vi "THz_TimeDelay.vi"(8 "error in (no error)":errorcluster, 11 "Transport":refnum<class "Transport.lvclass">) -> (0 "error out":errorcluster, 3 "Transport out":refnum<class "Transport.lvclass">)   [LabVIEW 2019, in "Transport.lvclass"]
uses:
  Transport.lvclass
  Transport.lvclass/Transport.ctl
  Control Experiment/Control Experiment.lvclass/Control Experiment.ctl
  <vilib>/PRIrvin/XY Utilities/subVIs/Waveform to XY (single).vi
  <vilib>/PRIrvin/XY Utilities/subVIs/Get X and Y (single).vi
  <userlib>/_MGI/Timing/MGI Wait/MGI Wait (U32).vi
  <vilib>/Waveform/WDTOps.llb/WDT Append Waveforms DBL.vi
  <vilib>/Waveform/WDTOps.llb/Waveform to XY Pairs.vi
  <vilib>/Waveform/WDTOps.llb/WDT Waveform to XY Pairs DBL.vi
  <vilib>/measure/maspectr.llb/FFT Power Spectrum and PSD for 1 Chan.vi
  Control Experiment/Control Experiment.lvclass
  <userlib>/LevyLab/Lockin-Multichannel/Instrument.Lockin/Instrument.Lockin.lvclass
  <userlib>/LevyLab/Instrument Framework/Instrument Types/Delay Line/Instrument.DelayLine.lvclass
  <userlib>/LevyLab/Instrument Framework/Instrument Types/Cryostat/Instrument.Cryostat.lvclass
  <vilib>/measure/NI_MAPro.lvlib
  <vilib>/PRIrvin/XY Utilities/xy_utilities.lvlib
  <userlib>/LevyLab/Instrument Framework/Instrument Types/Lockin/Instrument.LockinAPI.lvclass
  C:/Program Files (x86)/National Instruments/LabVIEW 2019/user.lib/LevyLab/Instrument Framework/Instrument Types/Lockin/Instrument.LockinAPI.lvclass
  C:/Program Files (x86)/National Instruments/LabVIEW 2019/user.lib/LevyLab/Instrument Framework/Instrument/Instrument.lvclass
  C:/Program Files (x86)/National Instruments/LabVIEW 2019/vi.lib/JKI/JKI SMO/SMO/SMO.lvclass
  <vilib>/measure/maresamp.llb/Resample Pair of Arrays (single shot).vi
panel:
  out "Horizontal Progress Bar":dbl(slide)=0.5013000000000001 scale=-0.5..0.5
  out "Signal vs Time":T1(graph)
  out "Delay vs Time":cluster{"Time":dbl[], "Delay":dbl[]}(graph)
  out "Power Spectrum":cluster{"f0":dbl, "df":dbl, "magnitude":dbl[]}[](graph) caption="Power spectrum of time domain signal"
  in  "stop":bool
  in  "Experiment Comments":string="describe only the experiment you're doing right now"
  in  "Experiment Folder":string="05 - folder name"
  out "Delay (ps)":dbl
  out "Elapsed Time (s)":u32
  out "T (mK)":dbl
  out "Refresh Time (ms)":u32
  in  "Sweep Time (s)":dbl=10.0 format="%#_3p"
  in  "Initial Wait (s)":u32=1
  in  "Delay End (ps)":dbl=0.5
  in  "Delay Start (ps)":dbl=-0.5
  in  "Fs (S/s)":dbl=1000.0 min=1000.0 max=204800.0 format="%#_13g"
  in  "Lockin Refresh (s)":dbl=2.0
  in  "Timeout (ms)":i32=1000
  out "Current State":string="Exit"
  # "Start"
  # "End"
  # "*** Folder and comments are only read if this VI is top level. If is is called from Sweep Control then the folder and comments come from Sweep Control.vi ***"
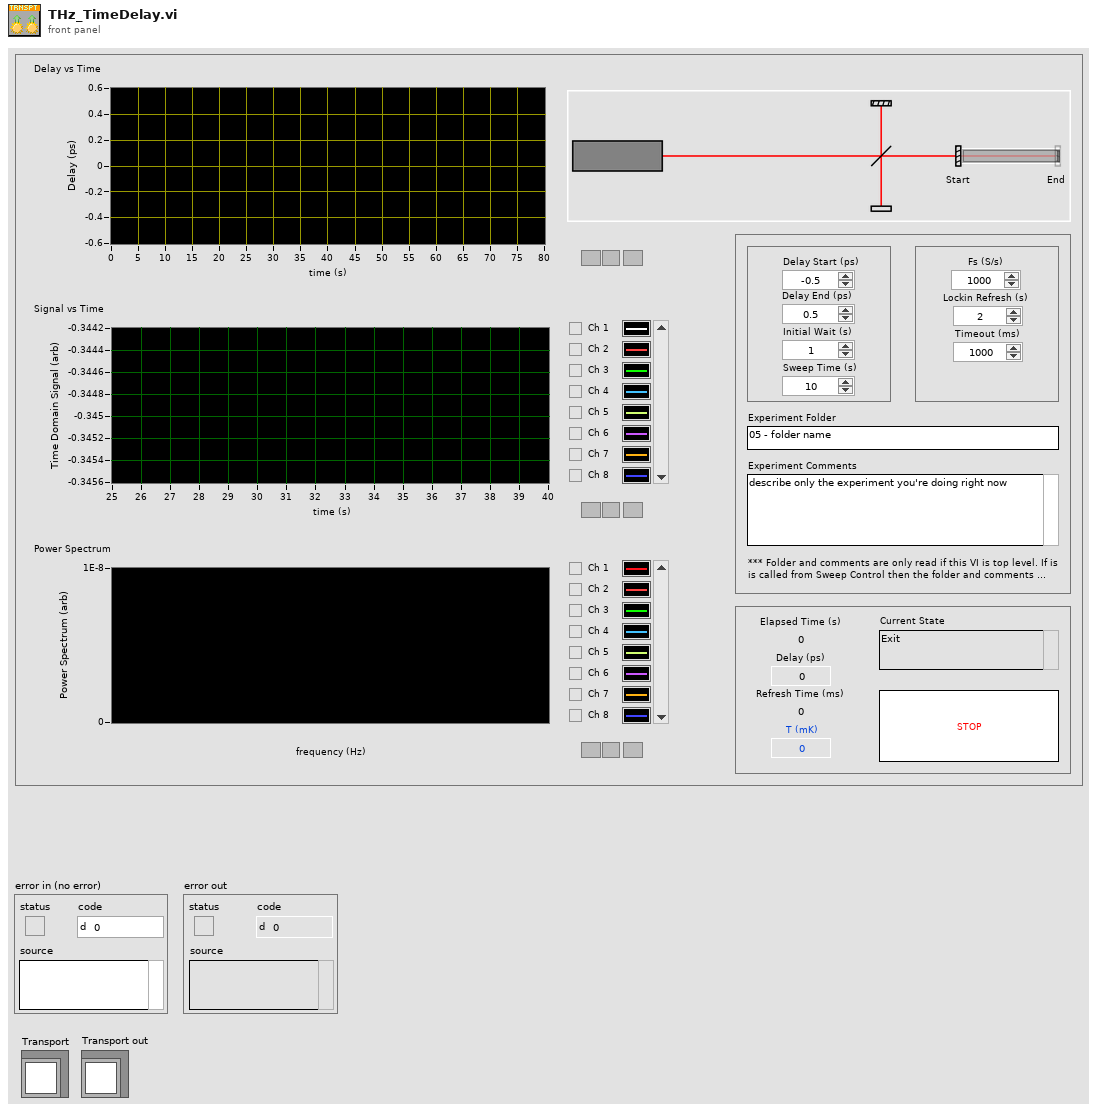
[diagram p1: front panel]
types:
  T1 = cluster{"Delay Start (ps)":dbl, dbl, "Y":dbl[]}[]
  T2 = enum32{"Invalid", "Standard", "Closed", "Hidden", "Minimized", "Maximized"}
  T3 = enum32{"invalid app kind", "Development System", "Run Time System", "Student Edition", "Embedded LabVIEW", "Evaluation", "Custom"}
  T4 = typedef "Control Experiment.lvclass/Instrument Classes--cluster.ctl" = cluster{"DAQ":refnum<class "Instrument.LockinAPI.lvclass">, "Amplifier":refnum<class "Instrument.Amplifier.lvclass">, "Temperature":refnum<class "Instrument.Cryostat.lvclass">, "Magnet":refnum<class "Instrument.Cryostat.lvclass">, "Rotator":refnum<class "Instrument.Cryostat.lvclass">, "Level":refnum<class "Instrument.Cryostat.lvclass">, "Capacitance":refnum<class "Instrument.CBridge.lvclass">, "Delay Line":refnum<class "Instrument.DelayLine.lvclass">, "Strain Cell":refnum<class "Instrument.Strain.lvclass">, "VNA":refnum<class "Instrument.VNA.lvclass">, "Source":refnum<class "Instrument.VSource.lvclass">}
  T5 = cluster{"Core":cluster{"Current VI Reference":refnum<vi>, "Close Panel on Exit?":bool}, "Transport":refnum<class "Transport.lvclass">, "C.E.":refnum<class "Control Experiment.lvclass">, "Instruments":T4, "Elapsed Time":dbl[], "Absolute Time":dbl[], "Temperature":dbl, "Magnet":dbl, "Delay":dbl[], "AI Waveform (s)":waveform(dbl)[], "AI Waveform (ps)":waveform(dbl)[], "t0":timestamp, "Sweep Value":dbl[], "ms [0]":u32, "ms [i]":u32, "Delay Range (ps)":dbl, "Delay Speed (ps/s)":dbl, "reset":bool, "delay line finish?":bool, "Execution:State":enum32{"Bad", "Idle", "Run top level", "Running"}}
  T6 = enum32{"Bad", "Idle", "Run top level", "Running"}
  T7 = cluster{"Current VI Reference":refnum<vi>, "Close Panel on Exit?":bool}
  T8 = typedef "Instrument.LockinAPI.lvclass/LockinAPI.Sampling.Sampling--Cluster.ctl" = cluster{"Fs":dbl, "#s":i32}
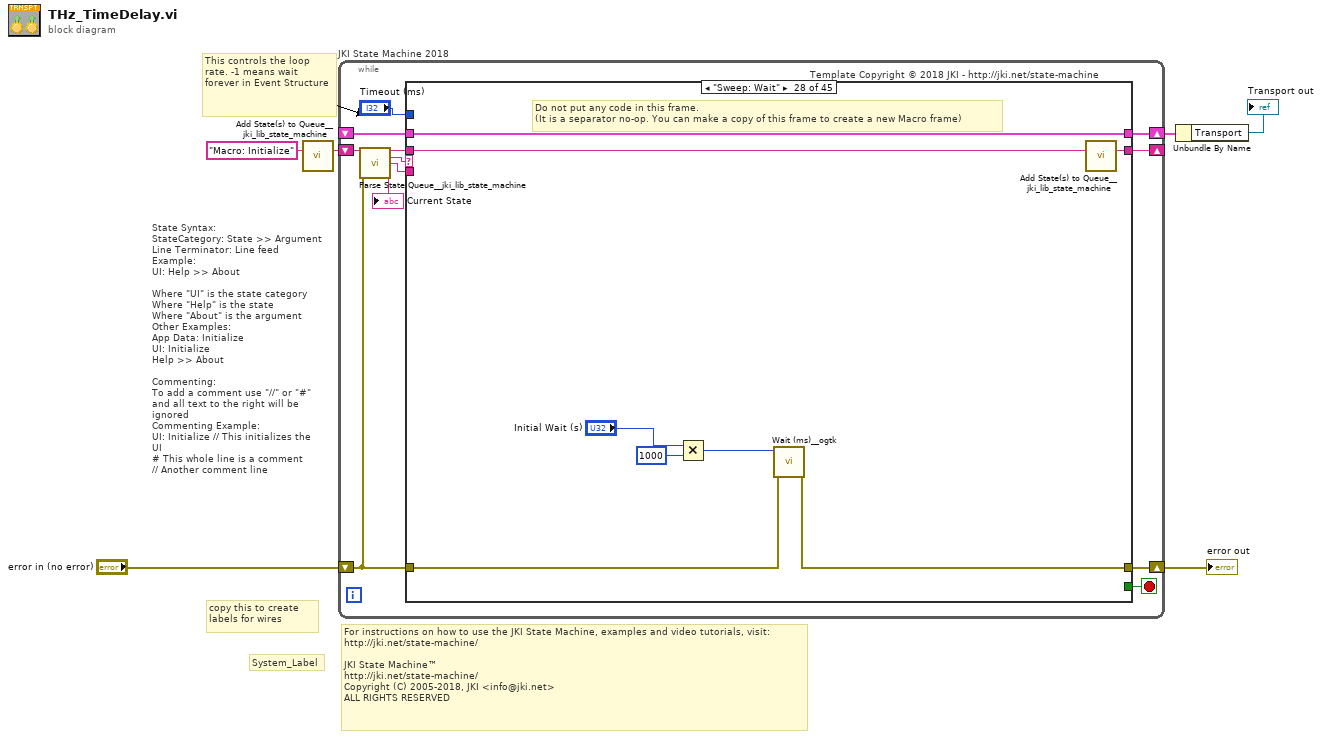
[diagram p0: block diagram]
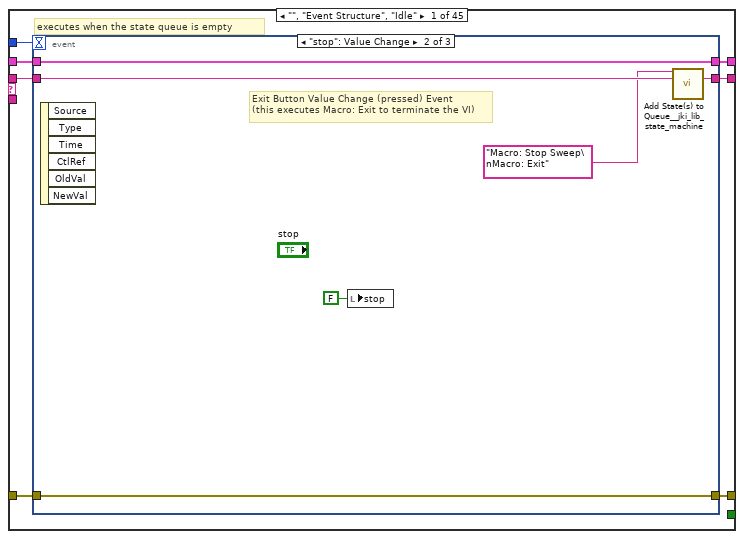
[diagram p2: hidden frame]
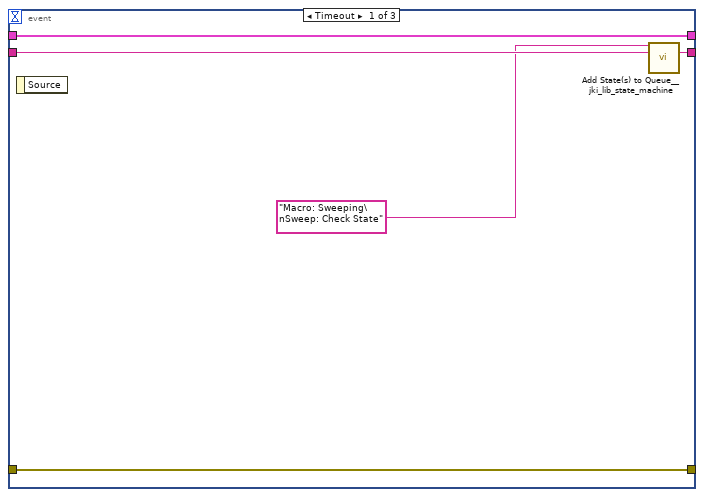
[diagram p3: hidden frame]
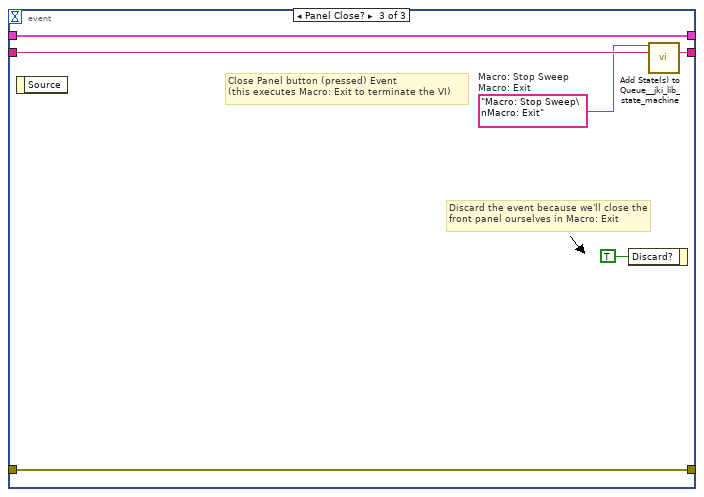
[diagram p4: hidden frame]
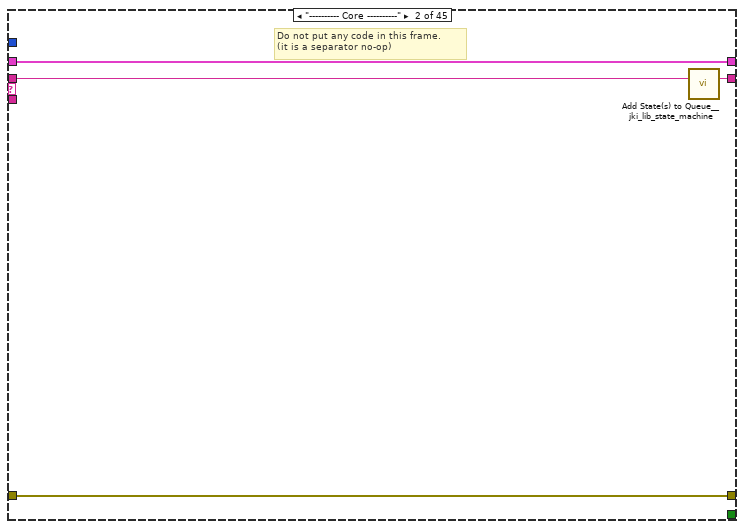
[diagram p5: hidden frame]
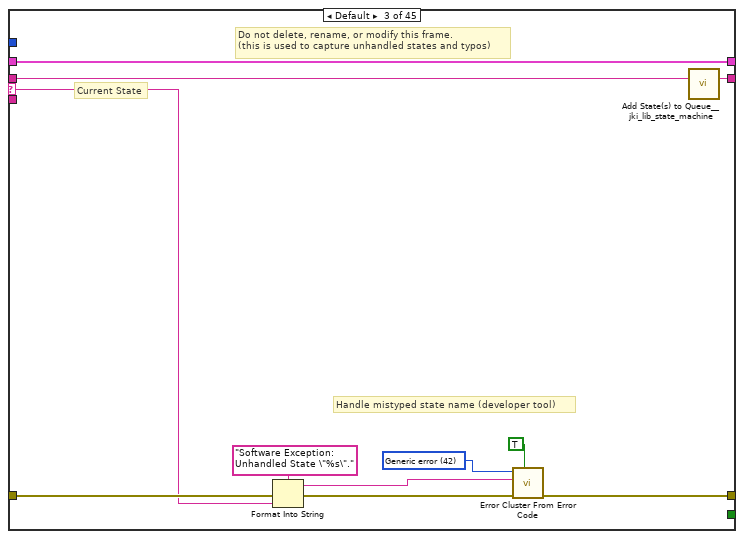
[diagram p6: hidden frame]
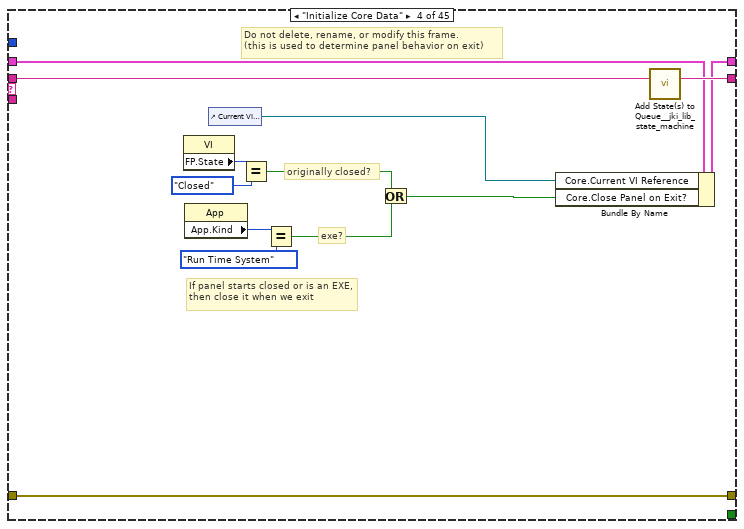
[diagram p7: hidden frame]
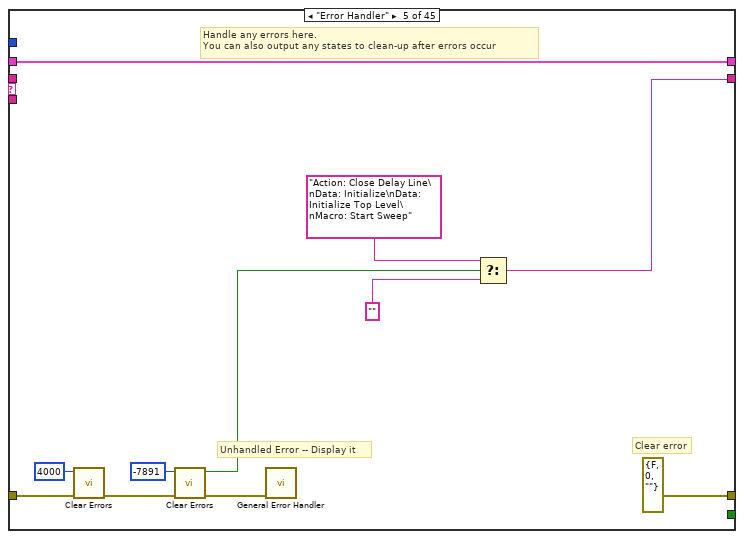
[diagram p8: hidden frame]
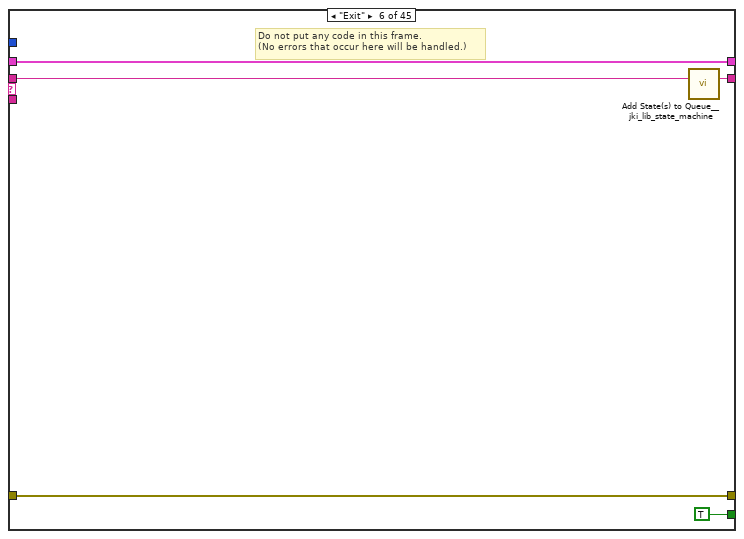
[diagram p9: hidden frame]
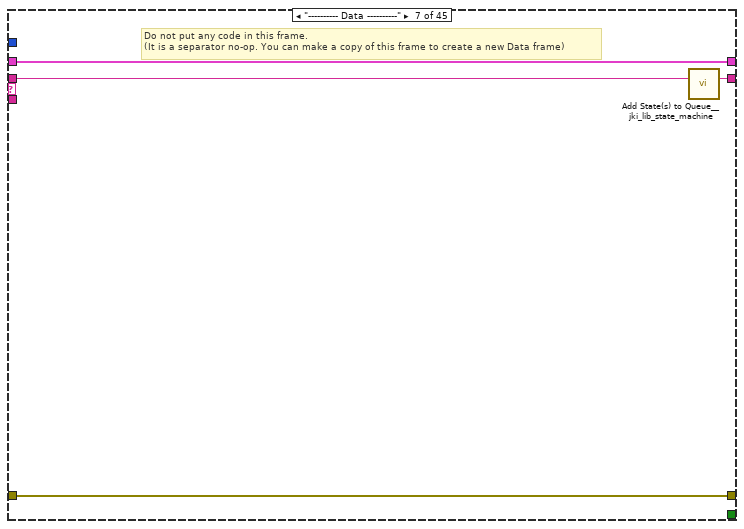
[diagram p10: hidden frame]
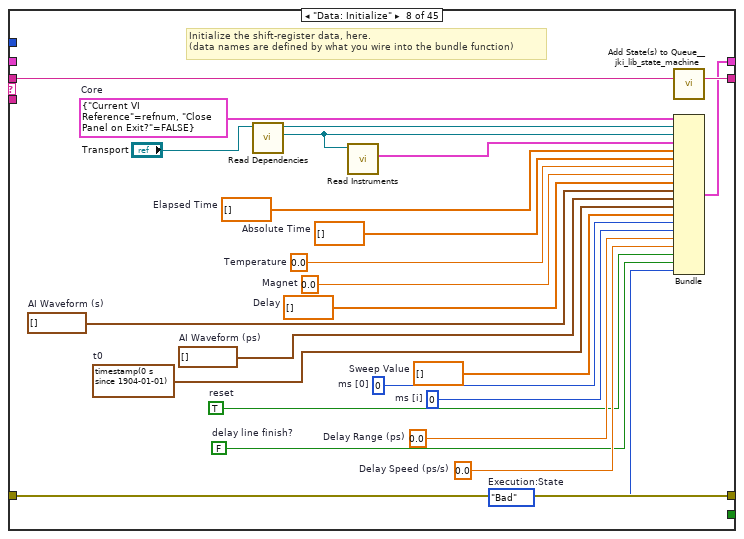
[diagram p11: hidden frame]
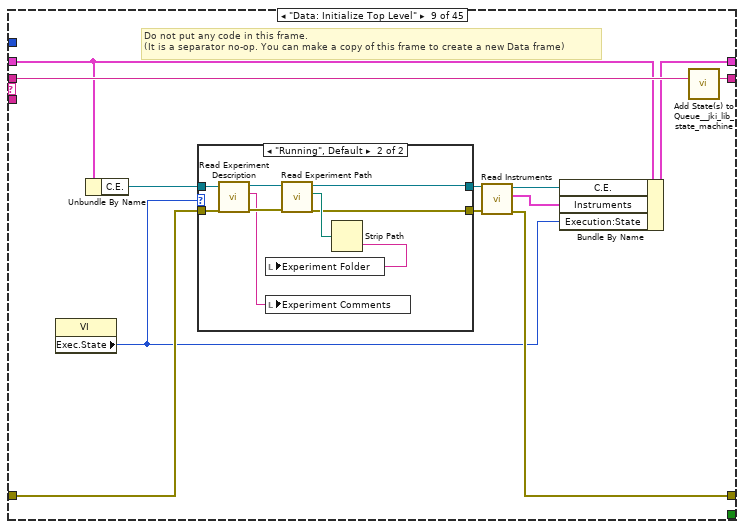
[diagram p12: hidden frame]
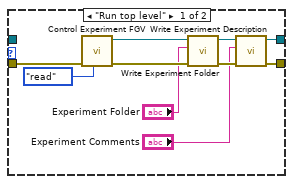
[diagram p13: hidden frame]
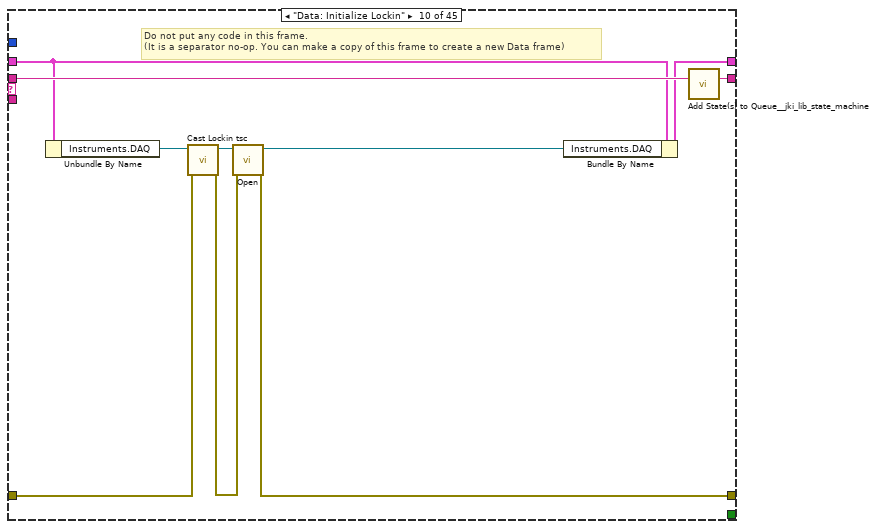
[diagram p14: hidden frame]
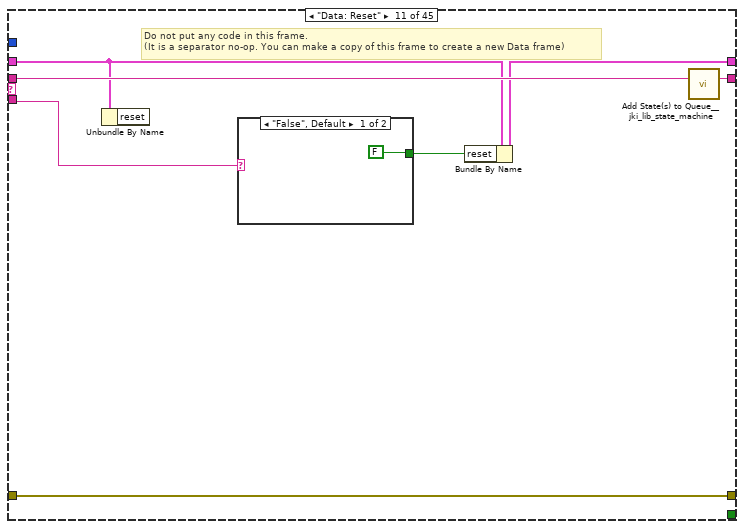
[diagram p15: hidden frame]
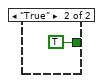
[diagram p16: hidden frame]
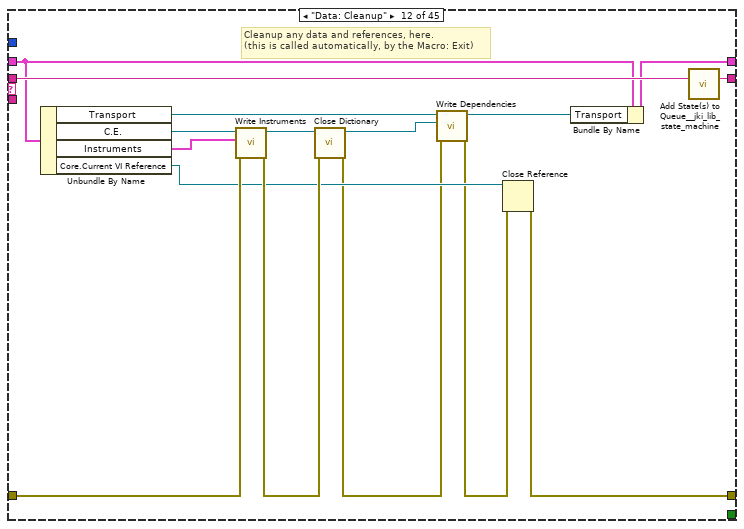
[diagram p17: hidden frame]
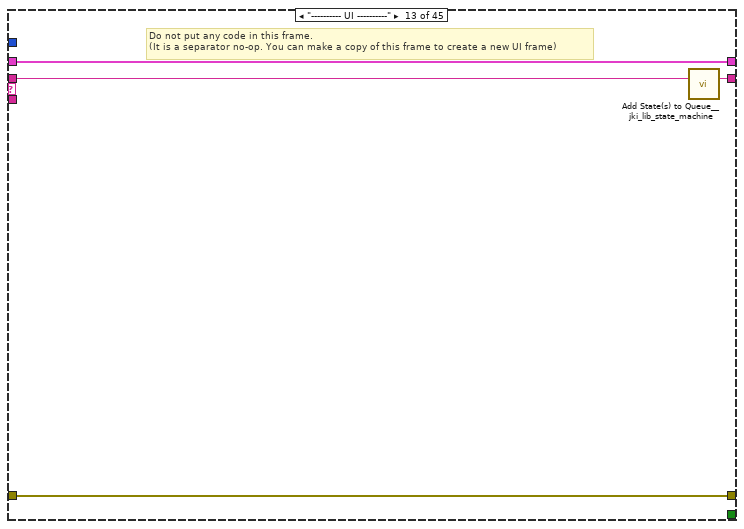
[diagram p18: hidden frame]
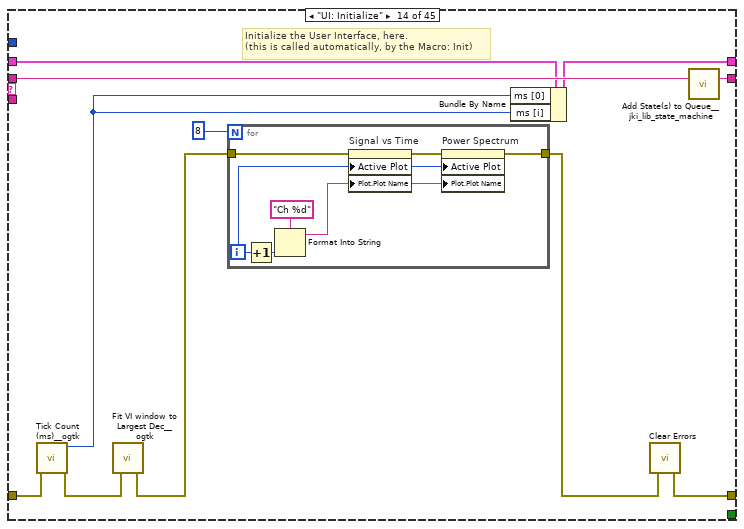
[diagram p19: hidden frame]
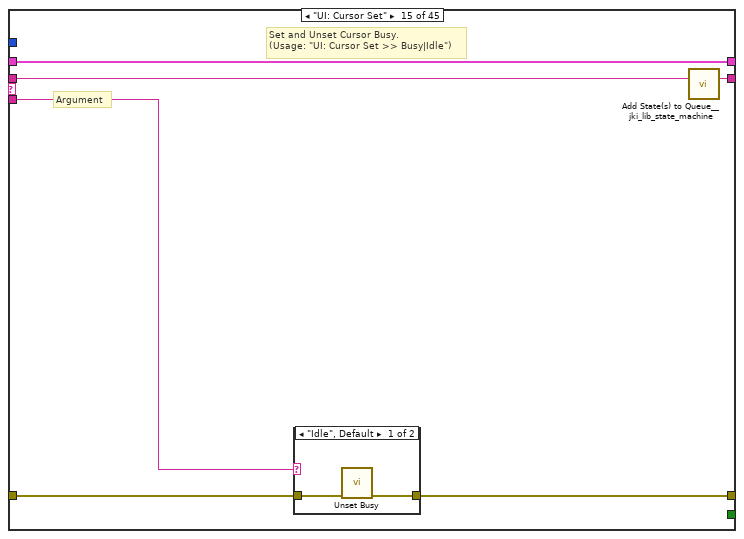
[diagram p20: hidden frame]
diagram:
  # "For instructions on how to use the JKI State Machine, examples and video tutorials, visit:\nhttp://jki.net/state-machine/\n\nJKI State Machine™\nhttp://jki.net/state-machine/\nCopyright (C) 2005-2018, JKI <info@jki.net>\nALL RIGHTS RESERVED"
  # "State Syntax:\nStateCategory: State >> Argument\nLine Terminator: Line feed\nExample:\nUI: Help >> About\n\nWhere \"UI\" is the state category\nWhere \"Help\" is the state\nWhere \"About\" is the argument\nOther Examples:\nApp Data: Initialize\nUI: Initialize\nHelp >> About\n\nCommenting:\nTo add a comment use \"//\" or \"#\" and all text to the right will be ignored\nCommenting Example:\nUI: Initialize // This initializes the UI\n# This whole line is a comment\n// Another comment line"
  # "copy this to create labels for wires"
  # "This controls the loop rate. -1 means wait forever in Event Structure"
  # "System_Label"
  n1 = call <vilib>:"Add State(s) to Queue__jki_lib_state_machine.vi"("State(s) in (\"\")"="Macro: Initialize") -> ("States Out"=w6:string)  [unwired: 14 in]
  n2 = while "JKI State Machine 2018" {
    shift-right: [w11] -> w4
    shift-left: _ -> [w10]
    shift-right: [w14] -> w3
    shift-left: "error in (no error)" -> [w8]
    shift-right: [w13] -> _
    shift-left: w6 -> [w15]
    stop <- w12 stop-if-true
    # "Template Copyright © 2018 JKI - http://jki.net/state-machine"
    n3 = call <vilib>:"Parse State Queue__jki_lib_state_machine.vi"("State Queue"=w15, "Error In (no error)"=w8) -> ("Remaining States"=w17:string, "Current State"=w7:string, "Arguments"=w16:string)  [unwired: 11 in]
    "Current State" <- w7
    n4 = case shown="\"Sweep: Wait\"" w7 {
      selector: w7 -> [_ _ w46 _ _ _ _ _ _ _ _ _ _ _ _ _ _ _ _ _ _ _ _ _ _ _ _ _ _ _ _ _ _ _ _ _ _ _ _ _ _ _ _ _ _]
      tunnel: w17 -> [w24 w45 w50 w69 _ w85 w89 w114 w126 w155 w162 w180 w184 w195 w208 w224 w247 w265 w272 w341 w349 w354 w359 w364 w374 w378 w392 w400 w404 w412 w417 w436 w445 w470 w489 w501 w505 w518 w577 w599 w617 w621 w625 w639 w684]
      tunnel: w16 -> [_ _ _ _ _ _ _ _ _ _ w157 _ _ _ w203 _ _ _ w266 _ _ _ _ _ _ _ _ _ _ _ _ _ w443 _ w486 _ _ w508 _ _ _ _ _ _ _]
      tunnel: w10 -> [w22 w42 w48 w62 w79 w83 w86 _ w118 w151 w159 w178 w181 w191 w206 w215 w237 w260 w268 w338 w347 w350 w356 w361 w371 w375 w379 w398 w402 w410 w414 w433 w439 w456 w478 w496 w502 w516 w573 w596 w615 w618 w622 w629 w682]
      tunnel: [w21 w43 w52 w66 errorcluster {"status"=FALSE, "code"=0, "source"=""} ("error out") w82 w87 w111 w119 w150 w160 w165 w182 w185 w204 w221 w239 w255 w269 w339 w346 w352 w357 w362 w372 w376 w384 w396 w401 w405 w415 w434 w440 w468 w481 w497 w503 w512 w567 w591 w606 w619 w623 w635 w681] -> w14
      tunnel: w8 -> [w20 w43 w51 w66 w77 w82 w87 w111 w120 w146 w160 w171 w182 w192 w205 w221 w240 w262 w270 w339 w346 w352 w357 w362 w372 w376 w388 w397 w401 w405 w415 w434 w441 w460 w482 w498 w503 w509 w574 w592 w607 w619 w623 w634 w681]
      tunnel: [w23 w44 w49 w68 w74 w84 w88 w113 w125 w154 w161 w179 w183 w194 w207 w223 w246 w264 w271 w340 w348 w353 w358 w363 w373 w377 w391 w399 w403 w411 w416 w435 w444 w469 w488 w500 w504 w517 w576 w598 w616 w620 w624 w638 w683] -> w13
      tunnel: [_ _ _ _ _ TRUE _ _ _ _ _ _ _ _ _ _ _ _ _ _ _ _ _ _ _ _ _ _ _ _ _ _ _ _ _ _ _ _ _ _ _ _ _ _ _] -> w12
      tunnel: [w19 w42 w48 w67 w79 w83 w86 w112 w117 w152 w158 w177 w181 w190 w206 w214 w237 w259 w268 w338 w347 w350 w356 w361 w371 w375 w390 w398 w402 w410 w414 w433 w437 w455 w479 w494 w502 w515 w572 w597 w614 w618 w622 w628 w682] -> w11
      tunnel: "Timeout (ms)" -> [w18 _ _ _ _ _ _ _ _ _ _ _ _ _ _ _ _ _ _ _ _ _ _ _ _ _ _ _ _ _ _ _ _ _ _ _ _ _ _ _ _ _ _ _ _]
      frame "", "Event Structure", "Idle" {
        # "executes when the state queue is empty"
        n5 = event shown="[1] \"stop\": Value Change" {
          selector: _ -> [_ _ _]
          dyn-events: _ -> [_ _ _]
          timeout: w18 -> [_ _ _]
          tunnel: w24 -> [w29 w35 w41]
          tunnel: [w28 w34 w40] -> w23
          tunnel: w22 -> [w26 w32 w38]
          tunnel: [w27 w33 w39] -> w21
          tunnel: w20 -> [w27 w33 w39]
          tunnel: [w26 w32 w38] -> w19
          event Timeout {
            n6 = event-data() -> ()  [unwired: 1 in, 1 out]
            n7 = call <vilib>:"Add State(s) to Queue__jki_lib_state_machine.vi"("State(s) in Front (\"\")"="Macro: Sweeping\nSweep: Check State" ("State(s) in Front (\"\")"), "State(s) in (\"\")"=w29) -> ("States Out"=w28:string)  [unwired: 13 in]
          }
          event "stop": Value Change {
            # "Exit Button Value Change (pressed) Event\n(this executes Macro: Exit to terminate the VI)"
            n8 = event-data() -> ()  [unwired: 1 in, 6 out]
            n9 = local write "stop"(FALSE ("stop")) -> ()
            n10 = call <vilib>:"Add State(s) to Queue__jki_lib_state_machine.vi"("State(s) in Front (\"\")"="Macro: Stop Sweep\nMacro: Exit", "State(s) in (\"\")"=w35) -> ("States Out"=w34:string)  [unwired: 13 in]
          }
          event Panel Close? {
            w37 = "Macro: Stop Sweep\nMacro: Exit"  # Macro: Stop Sweep Macro: Exit
            # "Discard the event because we'll close the front panel ourselves in Macro: Exit"
            # "Close Panel button (pressed) Event\n(this executes Macro: Exit to terminate the VI)"
            n11 = event-data() -> ()  [unwired: 1 in, 1 out]
            n12 = event-data("Discard?"=TRUE) -> ()  [unwired: 1 in, 1 out]
            n13 = call <vilib>:"Add State(s) to Queue__jki_lib_state_machine.vi"("State(s) in Front (\"\")"=w37, "State(s) in (\"\")"=w41) -> ("States Out"=w40:string)  [unwired: 13 in]
          }
        }
      }
      frame "---------- Core ----------" {
        # "Do not put any code in this frame.\n(it is a separator no-op)"
        n14 = call <vilib>:"Add State(s) to Queue__jki_lib_state_machine.vi"("State(s) in (\"\")"=w45) -> ("States Out"=w44:string)  [unwired: 14 in]
      }
      frame Default {
        w55 = 42 items=["No error", "Argument error", "Memory is full", "Out of zone", "End of file", "File already open", "Generic file I/O error", "File not found", "File permission error", "Disk is full", "Duplicate path", "Too many files open", "System feature not enabled", "Resource file not found", "Cannot add resource", "Resource not found", "Image not found", "Image memory error", "Pen does not exist", "Config type invalid", "Config token not found", "Config parse error", "Config memory error", "Bad external code format", "Bad external code offset", "External code not present", "Null window", "Destroy window error", "Null menu", "Print aborted", "Bad print record", "Print driver error", "Windows error during printing", "Memory error during printing", "Print dialog error", "Generic print error", "Invalid device refnum", "Device not found", "Device parameter error", "Device unit error", "Cannot open device", "Device call aborted", "Generic error", "Cancelled by user", "Object ID too low", "Object ID too high", "Object not in heap", "Unknown heap", "Unknown object (invalid DefProc)", "Unknown object (DefProc not in table)", "Message out of range", "Invalid (null) method", "Unknown message", "Manager call not supported", "Bad address", "Network operation in progress", "Network operation timed out", "Connection is busy", "Network attribute not supported", "Network error", "Address in use", "System out of memory", "Connection aborted", "Connection refused", "Not connected", "Already connected", "Connection closed", "Initialization error (interapplication manager)", "Bad occurrence", "Wait on unbound occurrence handler", "Occurrence queue overflow", "Datalog type conflict", "Unused", "Unrecognized type (interapplication manager)", "Memory corrupt", "Failed to make temporary DLL", "Old CIN version", "Drag socket not found", "Failed to load drop-object", "Failed to register OLE object", "Failed to release OLE object", "Format specifier type mismatch", "Unknown format specifier", "Too few format specifiers", "Too many format specifiers", "Scan failed", "Newer CIN version", "Error converting to variant", "Runtime menu error", "Password tampered", "Variant attribute not found", "Incompatible variant data type", "Event data is not available", "Event Store is not present", "Occurrence is not found", "Event Queue is not created", "Event info is not available", "Refnum passed is NULL", "Error retrieving Class GUID", "Error retrieving CoClass GUID", "Error retrieving TypeLib GUID.", "Bad built application magic bytes.", "Specific driver is different from the specific driver associated with the Logical Name.", "There is no session opened to the class driver.", "Max Error", "MAX - Error with config objects", "MAX - Error loading configuration", "MAX - Group not supported"]
        # "Current State"
        # "Do not delete, rename, or modify this frame.\n(this is used to capture unhandled states and typos)"
        # "Handle mistyped state name (developer tool)"
        n15 = Format Into String(format string="Software Exception: Unhandled State \"%s\"." ("message"), error in=w51, w46) -> (resulting string=w54:string, error out=w53:errorcluster)  [unwired: 1 in]
        n16 = call <vilib>:"Error Cluster From Error Code.vi"("show call chain? (False)"=TRUE, "error in (no error)"=w53, "error message (\"\")"=w54, "error code (0)"=w55) -> ("error out"=w52:errorcluster)  [unwired: 5 in]
        n17 = call <vilib>:"Add State(s) to Queue__jki_lib_state_machine.vi"("State(s) in (\"\")"=w50) -> ("States Out"=w49:string)  [unwired: 14 in]
      }
      frame "Initialize Core Data" {
        # "Do not delete, rename, or modify this frame.\n(this is used to determine panel behavior on exit)"
        # "originally closed?"
        # "exe?"
        # "If panel starts closed or is an EXE, then close it when we exit"
        n18 = property class="VI"() -> ("FP.State"=w59:T2)  [unwired: 2 in, 2 out]
        n19 = property class="App"() -> ("App.Kind"=w65:T3)  [unwired: 2 in, 2 out]
        n20 = control-ref of="Current VI Reference"() -> (w60:refnum<vi>)
        n21 = Equal?(x=w59, y=T2."Closed" ("Front Panel Window:State")) -> (x = y?=w57:bool)
        n22 = Equal?(x=w65, y=T3."Run Time System" ("Application:Kind")) -> (x = y?=w63:bool)
        n23 = Or(x=w57, y=w63) -> (x .or. y?=w61:bool)
        n24 = Bundle By Name(cluster=w62, "Core.Current VI Reference"=w60, "Core.Close Panel on Exit?"=w61) -> (w67:T5)
        n25 = call <vilib>:"Add State(s) to Queue__jki_lib_state_machine.vi"("State(s) in (\"\")"=w69) -> ("States Out"=w68:string)  [unwired: 14 in]
      }
      frame "Error Handler" {
        # "Unhandled Error -- Display it"
        # "Handle any errors here.\nYou can also output any states to clean-up after errors occur"
        # "Clear error"
        n26 = call <vilib>:"Clear Errors.vi"("error in (no error)"=w77, "specific error code to clear (0: all)"=4000) -> ("error out"=w72:errorcluster)  [unwired: 4 in, 1 out]
        n27 = call <vilib>:"Clear Errors.vi"("error in (no error)"=w72, "specific error code to clear (0: all)"=-7891) -> ("error out"=w71:errorcluster, "specific error cleared?"=w70:bool)  [unwired: 4 in]
        n28 = call <vilib>:"General Error Handler.vi"("error in (no error)"=w71) -> ()  [unwired: 10 in, 5 out]
        n29 = Select(t="Action: Close Delay Line\nData: Initialize\nData: Initialize Top Level\nMacro: Start Sweep", s=w70, f="") -> (s? t:f=w74:string)
      }
      frame "Exit" {
        # "Do not put any code in this frame.\n(No errors that occur here will be handled.)"
        n30 = call <vilib>:"Add State(s) to Queue__jki_lib_state_machine.vi"("State(s) in (\"\")"=w85) -> ("States Out"=w84:string)  [unwired: 14 in]
      }
      frame "---------- Data ----------" {
        # "Do not put any code in this frame.\n(It is a separator no-op. You can make a copy of this frame to create a new Data frame)"
        n31 = call <vilib>:"Add State(s) to Queue__jki_lib_state_machine.vi"("State(s) in (\"\")"=w89) -> ("States Out"=w88:string)  [unwired: 14 in]
      }
      frame "Data: Initialize" {
        w94 = T6."Bad"  # Execution:State
        w95 = waveform(dbl)[] []  # AI Waveform (ps)
        w96 = FALSE  # delay line finish?
        w97 = TRUE  # reset
        w102 = dbl[] []  # Absolute Time
        w98 = waveform(dbl)[] []  # AI Waveform (s)
        w104 = timestamp(0 s since 1904-01-01)  # t0
        w105 = 0.0  # Delay Speed (ps/s)
        w99 = dbl[] []  # Delay
        w106 = 0.0  # Delay Range (ps)
        w107 = dbl[] []  # Sweep Value
        w108 = u32 0  # ms [i]
        w109 = u32 0  # ms [0]
        w103 = dbl[] []  # Elapsed Time
        w100 = 0.0  # Magnet
        w101 = 0.0  # Temperature
        w110 = T7 {"Current VI Reference"=refnum, "Close Panel on Exit?"=FALSE}  # Core
        # "Initialize the shift-register data, here.\n(data names are defined by what you wire into the bundle function)"
        n32 = call "Read Dependencies.vi"("Transport"="Transport") -> ("C.E."=w91:refnum<class "Control Experiment.lvclass">, "Transport"=w92:refnum<class "Transport.lvclass">)  [unwired: 8 in, 1 out]
        n33 = call "Read Instruments.vi"("Control Experiment in"=w91) -> ("Instruments"=w90:T4)  [unwired: 8 in, 2 out]
        n34 = call <vilib>:"Add State(s) to Queue__jki_lib_state_machine.vi"("State(s) in (\"\")"=w114) -> ("States Out"=w113:string)  [unwired: 14 in]
        n35 = Bundle("Core"=w110, "Transport"=w92, "C.E."=w91, "Instruments"=w90, "Elapsed Time"=w103, "Absolute Time"=w102, "Temperature"=w101, "Magnet"=w100, "Delay"=w99, "AI Waveform (s)"=w98, "AI Waveform (ps)"=w95, "t0"=w104, "Sweep Value"=w107, "ms [0]"=w109, "ms [i]"=w108, "Delay Range (ps)"=w106, "Delay Speed (ps/s)"=w105, "reset"=w97, "delay line finish?"=w96, "Execution:State"=w94) -> (w112:T5)  [unwired: 1 in]
      }
      frame "Data: Initialize Top Level" {
        # "Do not put any code in this frame.\n(It is a separator no-op. You can make a copy of this frame to create a new Data frame)"
        n36 = property class="VI"() -> ("Exec.State"=w115:T6)  [unwired: 2 in, 2 out]
        n37 = Unbundle By Name(w118) -> ("C.E."=w121:refnum<class "Control Experiment.lvclass">)
        n38 = case shown="\"Running\", Default" w115 {
          tunnel: w120 -> [w136 w142]
          tunnel: [w131 w139] -> w122
          tunnel: [w130 w140] -> w123
          tunnel: w121 -> [_ w141]
          frame "Run top level" {
            n39 = call "Control Experiment FGV.vi"("Function"=enum16{"read", "write"}."read", "error in (no error)"=w136) -> ("error out"=w134:errorcluster, "Control Experiment.lvclass out"=w135:refnum<class "Control Experiment.lvclass">)  [unwired: 8 in]
            n40 = call "Write Experiment Folder.vi"("error in (no error)"=w134, "Experiment Folder"="Experiment Folder", "Control Experiment in"=w135) -> ("error out"=w132:errorcluster, "Control Experiment out"=w133:refnum<class "Control Experiment.lvclass">)  [unwired: 7 in]
            n41 = call "Write Experiment Description.vi"("error in (no error)"=w132, "Experiment Description"="Experiment Comments", "Control Experiment in"=w133) -> ("error out"=w131:errorcluster, "Control Experiment out"=w130:refnum<class "Control Experiment.lvclass">)  [unwired: 7 in]
          }
          frame "Running", Default {
            n42 = call "Read Experiment Description.vi"("error in (no error)"=w142, "Control Experiment in"=w141) -> ("error out"=w144:errorcluster, "Experiment Description"=w138:string, "Control Experiment out"=w143:refnum<class "Control Experiment.lvclass">)  [unwired: 7 in]
            n43 = local write "Experiment Comments"(w138) -> ()
            n44 = call "Read Experiment Path.vi"("error in (no error)"=w144, "Control Experiment in"=w143) -> ("error out"=w139:errorcluster, "Experiment Path"=w145:path, "Control Experiment out"=w140:refnum<class "Control Experiment.lvclass">)  [unwired: 7 in]
            n45 = Strip Path(path=w145) -> (name=w137:string)  [unwired: 1 out]
            n46 = local write "Experiment Folder"(w137) -> ()
          }
        }
        n47 = call "Read Instruments.vi"("error in (no error)"=w122, "Control Experiment in"=w123) -> ("error out"=w119:errorcluster, "Instruments"=w124:T4, "Control Experiment out"=w116:refnum<class "Control Experiment.lvclass">)  [unwired: 7 in]
        n48 = Bundle By Name(cluster=w118, "C.E."=w116, "Instruments"=w124, "Execution:State"=w115) -> (w117:T5)
        n49 = call <vilib>:"Add State(s) to Queue__jki_lib_state_machine.vi"("State(s) in (\"\")"=w126) -> ("States Out"=w125:string)  [unwired: 14 in]
      }
      frame "Data: Initialize Lockin" {
        # "Do not put any code in this frame.\n(It is a separator no-op. You can make a copy of this frame to create a new Data frame)"
        n50 = Unbundle By Name(w151) -> ("Instruments.DAQ"=w149:refnum<class "Instrument.LockinAPI.lvclass">)
        n51 = call "Cast Lockin tsc.vi"("error in (no error)"=w146, "Instrument.LockinAPI in"=w149) -> ("error out"=w147:errorcluster, "Instrument.Lockin out"=w148:refnum<class "Instrument.Lockin.lvclass">)  [unwired: 8 in]
        n52 = call-dynamic "Open.vi"("error in (no error)"=w147, "Instrument.Lockin in"=w148) -> ("error out"=w150:errorcluster, "Instrument.Lockin out"=w153:refnum<class "Instrument.Lockin.lvclass">)  [unwired: 8 in]
        n53 = Bundle By Name(cluster=w151, "Instruments.DAQ"=w153) -> (w152:T5)
        n54 = call <vilib>:"Add State(s) to Queue__jki_lib_state_machine.vi"("State(s) in (\"\")"=w155) -> ("States Out"=w154:string)  [unwired: 14 in]
      }
      frame "Data: Reset" {
        # "Do not put any code in this frame.\n(It is a separator no-op. You can make a copy of this frame to create a new Data frame)"
        n55 = Unbundle By Name(w159) -> ()  [unwired: 1 out]
        n56 = case shown="\"False\", Default" w157 {
          tunnel: [FALSE ("reset") TRUE ("reset")] -> w156
          frame "False", Default {
          }
          frame "True" {
          }
        }
        n57 = Bundle By Name(cluster=w159, "reset"=w156) -> (w158:T5)
        n58 = call <vilib>:"Add State(s) to Queue__jki_lib_state_machine.vi"("State(s) in (\"\")"=w162) -> ("States Out"=w161:string)  [unwired: 14 in]
      }
      frame "Data: Cleanup" {
        # "Cleanup any data and references, here.\n(this is called automatically, by the Macro: Exit)"
        n59 = Unbundle By Name(w178) -> ("Transport"=w175:refnum<class "Transport.lvclass">, "C.E."=w174:refnum<class "Control Experiment.lvclass">, "Instruments"=w172:T4, "Core.Current VI Reference"=w169:refnum<vi>)
        n60 = call "Write Instruments.vi"("error in (no error)"=w171, "Instruments"=w172, "Control Experiment in"=w174) -> ("error out"=w170:errorcluster, "Control Experiment out"=w173:refnum<class "Control Experiment.lvclass">)  [unwired: 7 in]
        n61 = call "Close Dictionary.vi"("error in (no error)"=w170, "Control Experiment in"=w173) -> ("error out"=w167:errorcluster, "Control Experiment out"=w168:refnum<class "Control Experiment.lvclass">)  [unwired: 8 in]
        n62 = call "Write Dependencies.vi"("error in (no error)"=w167, "Control Experiment"=w168, "Transport in"=w175) -> ("error out"=w166:errorcluster, "Transport out"=w176:refnum<class "Transport.lvclass">)  [unwired: 7 in]
        n63 = Close Reference(reference=w169, error in (no error)=w166) -> (error out=w165:errorcluster)
        n64 = Bundle By Name(cluster=w178, "Transport"=w176) -> (w177:T5)
        n65 = call <vilib>:"Add State(s) to Queue__jki_lib_state_machine.vi"("State(s) in (\"\")"=w180) -> ("States Out"=w179:string)  [unwired: 14 in]
      }
      frame "---------- UI ----------" {
        # "Do not put any code in this frame.\n(It is a separator no-op. You can make a copy of this frame to create a new UI frame)"
        n66 = call <vilib>:"Add State(s) to Queue__jki_lib_state_machine.vi"("State(s) in (\"\")"=w184) -> ("States Out"=w183:string)  [unwired: 14 in]
      }
      frame "UI: Initialize" {
        # "Initialize the User Interface, here.\n(this is called automatically, by the Macro: Init)"
        n67 = call <userlib>:"Tick Count (ms)__ogtk.vi"("error in (no error)"=w192) -> ("error out"=w188:errorcluster, "millisecond timer value"=w189:u32)  [unwired: 9 in]
        n68 = call <userlib>:"Fit VI window to Largest Dec__ogtk.vi"("error in (no error)"=w188) -> ("error out"=w187:errorcluster)  [unwired: 5 in, 1 out]
        n69 = for {
          N: 8 -> [_]
          tunnel: w187 -> [w201]
          tunnel: [w197] -> w186
          i -> [w198]
          n70 = Increment(x=w198) -> (x+1=w200:i32)
          n71 = Format Into String(format string="Ch %d", w200) -> (resulting string=w196:string)  [unwired: 2 in, 1 out]
          n72 = property on="Signal vs Time" class="WFGraph (strict)"(error in=w201, "Active Plot"=w198, "Plot.Plot Name"=w196) -> (error out=w199:errorcluster)  [unwired: 1 in, 1 out]
          n73 = property on="Power Spectrum" class="WFGraph (strict)"(error in=w199, "Active Plot"=w198, "Plot.Plot Name"=w196) -> (error out=w197:errorcluster)  [unwired: 1 in, 1 out]
        }
        n74 = Bundle By Name(cluster=w191, "ms [0]"=w189, "ms [i]"=w189) -> (w190:T5)
        n75 = call <vilib>:"Clear Errors.vi"("error in (no error)"=w186) -> ("error out"=w185:errorcluster)  [unwired: 5 in, 1 out]
        n76 = call <vilib>:"Add State(s) to Queue__jki_lib_state_machine.vi"("State(s) in (\"\")"=w195) -> ("States Out"=w194:string)  [unwired: 14 in]
      }
      frame "UI: Cursor Set" {
        # "Argument"
        # "Set and Unset Cursor Busy.\n(Usage: \"UI: Cursor Set >> Busy|Idle\")"
        n77 = case shown="\"Idle\", Default" w203 {
          tunnel: w205 -> [w210 w212]
          tunnel: [w209 w211] -> w204
          frame "Idle", Default {
            n78 = call <vilib>:"Unset Busy.vi"("error in (no error)"=w210) -> ("error out"=w209:errorcluster)  [unwired: 10 in]
          }
          frame "Busy" {
            n79 = call <vilib>:"Set Busy.vi"("error in (no error)"=w212) -> ("error out"=w211:errorcluster)  [unwired: 9 in, 1 out]
          }
        }
        n80 = call <vilib>:"Add State(s) to Queue__jki_lib_state_machine.vi"("State(s) in (\"\")"=w208) -> ("States Out"=w207:string)  [unwired: 14 in]
      }
      frame "UI: Update Graphs" {
        # "Do not put any code in this frame.\n(It is a separator no-op. You can make a copy of this frame to create a new UI frame)"
        n81 = Unbundle By Name(w215) -> ("Elapsed Time"=w222:dbl[], "Delay"=w220:dbl[], "AI Waveform (s)"=w218:waveform(dbl)[], "Delay Speed (ps/s)"=w216:dbl)  [unwired: 1 out]
        n82 = Bundle("Elapsed Time"=w222, "Delay"=w220) -> (→"Delay vs Time":cluster{"Elapsed Time":dbl[], "Delay":dbl[]})  [unwired: 1 in]
        n83 = for {
          tunnel: w218 -> [w226] mode=indexing
          tunnel: [w228] -> w217 mode=indexing
          tunnel: w216 -> [w227]
          tunnel: [w225] -> w213 mode=indexing
          # "dt in ps"
          # "ps/s"
          # "dt in seconds"
          n84 = Unbundle By Name(w226) -> ("dt"=w232:dbl, "Y"=w230:dbl[])
          n85 = local read "Delay Start (ps)"() -> (w229:dbl)
          n86 = Multiply(x=w232, y=w227) -> (x*y=w231:dbl)
          n87 = Bundle By Name(cluster=w226, "dt"=w227) -> (w225:waveform(dbl))
          n88 = Bundle("Delay Start (ps)"=w229, w231, "Y"=w230) -> (w228:cluster{"Delay Start (ps)":dbl, dbl, "Y":dbl[]})  [unwired: 1 in]
        }
        "Signal vs Time" <- w217
        n89 = Bundle By Name(cluster=w215, "AI Waveform (ps)"=w213) -> (w214:T5)
        n90 = call <vilib>:"Add State(s) to Queue__jki_lib_state_machine.vi"("State(s) in (\"\")"=w224) -> ("States Out"=w223:string)  [unwired: 14 in]
      }
      frame "UI: Update Graphs Final" {
        # "Do not put any code in this frame.\n(It is a separator no-op. You can make a copy of this frame to create a new UI frame)"
        n91 = Unbundle By Name(w237) -> ("Absolute Time"=w235:dbl[], "Elapsed Time"=w242:dbl[], "Delay"=w236:dbl[], "AI Waveform (s)"=w233:waveform(dbl)[])
        n92 = Index Array(array=w233) -> (element=w245:waveform(dbl))  [unwired: 1 in]
        n93 = Bundle("Elapsed Time"=w242, "Delay"=w236) -> ()  [unwired: 1 in, 1 out]
        n94 = Unbundle By Name(w245) -> ("dt"=w244:dbl, "t0"=w243:timestamp)
        n95 = Bundle("Absolute Time"=w235, "Delay"=w236) -> (w234:cluster{"Absolute Time":dbl[], "Delay":dbl[]})  [unwired: 1 in]
        n96 = To Double Precision Float(number=w243) -> (double precision float=w241:dbl)
        n97 = call-poly <vilib>:"Resample Waveforms (single shot).vi"("XY-data in"=w234, "dt"=w244, "t0"=w241, "error in (no error)"=w240) -> ("resampled waveform out"=w238:waveform(dbl), "error out"=w239:errorcluster)  [unwired: 7 in, 3 out]
        n98 = for {
          tunnel: w238 -> [w252]
          tunnel: w233 -> [w251] mode=indexing
          tunnel: [w248] -> _ mode=indexing
          n99 = Unbundle By Name(w252) -> ("Y"=w250:dbl[])
          n100 = Unbundle By Name(w251) -> ("Y"=w249:dbl[])
          n101 = Bundle("Y"=w250, "Y"=w249) -> (w248:cluster{"Y":dbl[], "Y":dbl[]})  [unwired: 1 in]
        }
        n102 = call <vilib>:"Add State(s) to Queue__jki_lib_state_machine.vi"("State(s) in (\"\")"=w247) -> ("States Out"=w246:string)  [unwired: 14 in]
      }
      frame "UI: Update Timer" {
        n103 = Unbundle By Name(w260) -> ("ms [0]"=w261:u32)
        n104 = call <userlib>:"Tick Count (ms)__ogtk.vi"("error in (no error)"=w262) -> ("error out"=w256:errorcluster, "millisecond timer value"=w254:u32)  [unwired: 9 in]
        n105 = Subtract(x=w254, y=w261) -> (x-y=w258:u32)
        n106 = call <userlib>:"MGI Milliseconds Since Last Call.vi"("Error In"=w256) -> ("ms"=→"Refresh Time (ms)":u32, "Error Out"=w255:errorcluster)  [unwired: 5 in]
        n107 = Divide(x=w258, y=u32 1000 ("x")) -> (x/y=→"Elapsed Time (s)":dbl)
        n108 = Bundle By Name(cluster=w260, "ms [i]"=w254) -> (w259:T5)
        n109 = call <vilib>:"Add State(s) to Queue__jki_lib_state_machine.vi"("State(s) in (\"\")"=w265) -> ("States Out"=w264:string)  [unwired: 14 in]
      }
      frame "UI: Front Panel State" {
        # "Argument"
        # "Set Front Panel Open or Closed\n(Usage: \"UI: Front Panel State >> Open|Close\")"
        n110 = Unbundle By Name(w268) -> ("Core.Current VI Reference"=w267:refnum<vi>)
        n111 = case shown="\"Open\", \"Standard\", Default" w266 {
          tunnel: w270 -> [w278 w293 w304 w317 w330]
          tunnel: [w280 w294 w306 w319 w332] -> w269
          tunnel: w267 -> [w279 w291 w305 w318 w331]
          frame "Open", "Standard", Default {
            w273 = T2."Standard" ("State")
            n112 = property class="VI"(reference=w279, error in=w278) -> (reference out=w276:refnum<vi>, error out=w277:errorcluster, "FP.State"=w275:T2)
            n113 = Not Equal?(x=w275, y=w273) -> (x != y?=w274:bool)
            n114 = case shown="False" w274 {
              tunnel: [w284 w286] -> w280
              tunnel: w277 -> [w283 w286]
              tunnel: w276 -> [w282 _]
              tunnel: w273 -> [w281 _]
              frame True {
                n115 = invoke class="VI" method="FP.Open"(reference=w282, error in=w283, "Activate"=TRUE, "State"=w281) -> (error out=w284:errorcluster)  [unwired: 1 in, 4 out]
              }
              frame False {
              }
            }
          }
          frame "Close", "Closed" {
            n116 = property class="VI"(reference=w291, error in=w293) -> (reference out=w290:refnum<vi>, error out=w292:errorcluster, "FP.State"=w288:T2)
            n117 = Not Equal?(x=w288, y=T2."Closed" ("Front Panel Window:State")) -> (x != y?=w287:bool)
            n118 = case shown="True" w287 {
              tunnel: [w295 w298] -> w294
              tunnel: w292 -> [w295 w297]
              tunnel: w290 -> [_ w296]
              frame False {
              }
              frame True {
                n119 = invoke class="VI" method="FP.Close"(reference=w296, error in=w297) -> (error out=w298:errorcluster)  [unwired: 1 in, 2 out]
              }
            }
          }
          frame "Hidden", "Hide" {
            w299 = T2."Hidden" ("State")
            n120 = property class="VI"(reference=w305, error in=w304) -> (reference out=w302:refnum<vi>, error out=w303:errorcluster, "FP.State"=w301:T2)
            n121 = Not Equal?(x=w301, y=w299) -> (x != y?=w300:bool)
            n122 = case shown="True" w300 {
              tunnel: [w310 w311] -> w306
              tunnel: w303 -> [w309 w311]
              tunnel: w302 -> [w308 _]
              tunnel: w299 -> [w307 _]
              frame True {
                n123 = invoke class="VI" method="FP.Open"(reference=w308, error in=w309, "State"=w307) -> (error out=w310:errorcluster)  [unwired: 2 in, 4 out]
              }
              frame False {
              }
            }
          }
          frame "Minimize", "Minimized" {
            w312 = T2."Minimized" ("State")
            n124 = property class="VI"(reference=w318, error in=w317) -> (reference out=w315:refnum<vi>, error out=w316:errorcluster, "FP.State"=w314:T2)
            n125 = Not Equal?(x=w314, y=w312) -> (x != y?=w313:bool)
            n126 = case shown="True" w313 {
              tunnel: [w323 w324] -> w319
              tunnel: w316 -> [w322 w324]
              tunnel: w315 -> [w321 _]
              tunnel: w312 -> [w320 _]
              frame True {
                n127 = invoke class="VI" method="FP.Open"(reference=w321, error in=w322, "State"=w320) -> (error out=w323:errorcluster)  [unwired: 2 in, 4 out]
              }
              frame False {
              }
            }
          }
          frame "Maximize", "Maximized" {
            w325 = T2."Maximized" ("State")
            n128 = property class="VI"(reference=w331, error in=w330) -> (reference out=w328:refnum<vi>, error out=w329:errorcluster, "FP.State"=w327:T2)
            n129 = Not Equal?(x=w327, y=w325) -> (x != y?=w326:bool)
            n130 = case shown="True" w326 {
              tunnel: [w336 w337] -> w332
              tunnel: w329 -> [w335 w337]
              tunnel: w328 -> [w334 _]
              tunnel: w325 -> [w333 _]
              frame True {
                n131 = invoke class="VI" method="FP.Open"(reference=w334, error in=w335, "State"=w333) -> (error out=w336:errorcluster)  [unwired: 2 in, 4 out]
              }
              frame False {
              }
            }
          }
        }
        n132 = call <vilib>:"Add State(s) to Queue__jki_lib_state_machine.vi"("State(s) in (\"\")"=w272) -> ("States Out"=w271:string)  [unwired: 14 in]
      }
      frame "---------- Macro ----------" {
        # "Do not put any code in this frame.\n(It is a separator no-op. You can make a copy of this frame to create a new Macro frame)"
        n133 = call <vilib>:"Add State(s) to Queue__jki_lib_state_machine.vi"("State(s) in (\"\")"=w341) -> ("States Out"=w340:string)  [unwired: 14 in]
      }
      frame "Macro: Initialize" {
        w344 = FALSE  # debug mode
        w343 = "Data: Initialize\nInitialize Core Data\nUI: Initialize\nUI: Front Panel State >> Open\nUI: Front Panel State >> Open\nData: Initialize Top Level\nData: Initialize Lockin\nData: Reset >> True\nSweep: Initialize\nSweep: Simulate\nMacro: Exit"  # debug mode
        # "Initialization Macro\n(This is called once, when the VI starts)"
        n134 = Select(t=w343, s=w344, f="Data: Initialize\nInitialize Core Data\nUI: Initialize\nUI: Front Panel State >> Open\nData: Initialize Top Level\nData: Reset >> True\nMacro: Start Sweep\n") -> (s? t:f=w345:string)
        n135 = call <vilib>:"Add State(s) to Queue__jki_lib_state_machine.vi"("State(s) in Front (\"\")"=w345, "State(s) in (\"\")"=w349) -> ("States Out"=w348:string)  [unwired: 13 in]
      }
      frame "Macro: Start Sweep" {
        # "Do not put any code in this frame.\n(It is a separator no-op. You can make a copy of this frame to create a new Macro frame)"
        n136 = call <vilib>:"Add State(s) to Queue__jki_lib_state_machine.vi"("State(s) in Front (\"\")"="Sweep: Initialize\nAction: Move Delay Line >> Start\n//Action: Lockin >> Stop\nAction: Lockin Sampling\nSweep: Wait\nMeasure: Lockin >> Start\n//Action: Lockin >> Start\nMeasure: Delay Line\nAction: Move Delay Line >> End" ("State(s) in Front (\"\")"), "State(s) in (\"\")"=w354) -> ("States Out"=w353:string)  [unwired: 13 in]
      }
      frame "Macro: Sweeping" {
        # "Do not put any code in this frame.\n(It is a separator no-op. You can make a copy of this frame to create a new Macro frame)"
        n137 = call <vilib>:"Add State(s) to Queue__jki_lib_state_machine.vi"("State(s) in Front (\"\")"="Measure: Lockin\n//Measure: Temperature\nMeasure: Time\nMeasure: Delay Line\nUI: Update Graphs\nUI: Update Timer\nData: Reset >> False" ("State(s) in Front (\"\")"), "State(s) in (\"\")"=w359) -> ("States Out"=w358:string)  [unwired: 13 in]
      }
      frame "Macro: Stop Sweep" {
        # "Do not put any code in this frame.\n(It is a separator no-op. You can make a copy of this frame to create a new Macro frame)"
        n138 = call <vilib>:"Add State(s) to Queue__jki_lib_state_machine.vi"("State(s) in Front (\"\")"="//Sweep: Stop\nUI: Update Graphs Final\nFile: Save\n//Action: Lockin >> Stop" ("State(s) in Front (\"\")"), "State(s) in (\"\")"=w364) -> ("States Out"=w363:string)  [unwired: 13 in]
      }
      frame "Macro: Exit" {
        # "Exit Macro\n(This is called once, when the VI exits)"
        n139 = Unbundle By Name(w371) -> ("Core.Close Panel on Exit?"=w370:bool)
        n140 = Select(t="UI: Front Panel State >> Close", s=w370, f="") -> (s? t:f=w367:string)
        n141 = call <vilib>:"Add State(s) to Queue__jki_lib_state_machine.vi"("State(s) in (\"\")"=w367, "State(s) at Back (\"\")"="Data: Cleanup\nExit") -> ("States Out"=w365:string)  [unwired: 13 in]
        n142 = call <vilib>:"Add State(s) to Queue__jki_lib_state_machine.vi"("State(s) in Front (\"\")"=w365, "State(s) in (\"\")"=w374) -> ("States Out"=w373:string)  [unwired: 13 in]
      }
      frame "---------- Sweep ----------" {
        # "Do not put any code in this frame.\n(It is a separator no-op. You can make a copy of this frame to create a new Macro frame)"
        n143 = call <vilib>:"Add State(s) to Queue__jki_lib_state_machine.vi"("State(s) in (\"\")"=w378) -> ("States Out"=w377:string)  [unwired: 14 in]
      }
      frame "Sweep: Initialize" {
        # "Do not put any code in this frame.\n(It is a separator no-op. You can make a copy of this frame to create a new Macro frame)"
        n144 = Unbundle By Name(w379) -> ("Instruments.Delay Line"=w389:refnum<class "Instrument.DelayLine.lvclass">)
        n145 = call-dynamic "Open.vi"("error in (no error)"=w388, "Instrument in"=w389) -> ("error out"=w384:errorcluster, "Instrument out"=w387:refnum<class "Instrument.DelayLine.lvclass">)  [unwired: 8 in]
        n146 = Subtract(x="Delay End (ps)", y="Delay Start (ps)") -> (x-y=w386:dbl)
        n147 = Absolute Value(x=w386) -> (abs(x)=w383:dbl)
        n148 = Divide(x=w383, y="Sweep Time (s)") -> (x/y=w385:dbl)
        n149 = Bundle By Name(cluster=w379, "Instruments.Delay Line"=w387, "Delay Range (ps)"=w383, "Delay Speed (ps/s)"=w385) -> (w390:T5)
        n150 = property on="Horizontal Progress Bar" class="Slide (strict)"("Scale.Maximum"="Delay End (ps)", "Scale.Minimum"="Delay Start (ps)") -> ()  [unwired: 2 in, 2 out]
        n151 = call <vilib>:"Add State(s) to Queue__jki_lib_state_machine.vi"("State(s) in (\"\")"=w392) -> ("States Out"=w391:string)  [unwired: 14 in]
      }
      frame "Sweep: Wait" {
        # "Do not put any code in this frame.\n(It is a separator no-op. You can make a copy of this frame to create a new Macro frame)"
        n152 = Multiply(x="Initial Wait (s)", y=u32 1000) -> (x*y=w394:u32)
        n153 = call <userlib>:"Wait (ms)__ogtk.vi"("error in (no error)"=w397, "milliseconds to wait"=w394) -> ("error out"=w396:errorcluster)  [unwired: 8 in, 1 out]
        n154 = call <vilib>:"Add State(s) to Queue__jki_lib_state_machine.vi"("State(s) in (\"\")"=w400) -> ("States Out"=w399:string)  [unwired: 14 in]
      }
      frame "Sweep: Stop" {
        # "#todo: is there a method to abort acquisition?"
        # "Do not put any code in this frame.\n(It is a separator no-op. You can make a copy of this frame to create a new Macro frame)"
        n155 = Unbundle By Name(w402) -> ()  [unwired: 1 out]
        n156 = call <vilib>:"Add State(s) to Queue__jki_lib_state_machine.vi"("State(s) in (\"\")"=w404) -> ("States Out"=w403:string)  [unwired: 14 in]
      }
      frame "Sweep: Check State" {
        # "Do not put any code in this frame.\n(It is a separator no-op. You can make a copy of this frame to create a new Macro frame)"
        n157 = Unbundle By Name(w410) -> ("delay line finish?"=w409:bool)
        n158 = Select(t="Macro: Sweeping\nMacro: Stop Sweep\nMacro: Exit" ("State(s) in Front (\"\")"), s=w409, f="") -> (s? t:f=w406:string)
        n159 = call <vilib>:"Add State(s) to Queue__jki_lib_state_machine.vi"("State(s) in Front (\"\")"=w406, "State(s) in (\"\")"=w412) -> ("States Out"=w411:string)  [unwired: 13 in]
      }
      frame "Sweep: Simulate" {
        # "Do not put any code in this frame.\n(It is a separator no-op. You can make a copy of this frame to create a new Macro frame)"
        n160 = Unbundle By Name(w414) -> ("Delay Speed (ps/s)"=w413:dbl)  [unwired: 1 out]
        n161 = while {
          tunnel: w413 -> [w427]
          i -> [w432]
          stop <- w430 stop-if-true
          n162 = Equal To 0?(x=w432) -> (x = 0?=w431:bool)
          n163 = local read "Delay Start (ps)"() -> (w429:dbl)
          n164 = call <userlib>:"MGI Milliseconds Since Last Reset.vi"("Reset (F)"=w431) -> ("ms"=w426:u32, "Error Out"=w420:errorcluster)  [unwired: 5 in]
          n165 = local read "Sweep Time (s)"() -> (w425:dbl)
          n166 = Divide(x=w426, y=1000.0) -> (x/y=w422:dbl)
          n167 = Multiply(x=w427, y=w422) -> (x*y=w423:dbl)
          n168 = call <userlib>:"MGI Milliseconds Since Last Call.vi"("Error In"=w420) -> ("ms"=w418:u32, "Error Out"=w419:errorcluster)  [unwired: 5 in]
          n169 = Add(x=w429, y=w423) -> (x+y=w428:dbl)
          n170 = local write "Elapsed Time (s)"(w422) -> ()
          n171 = Greater?(x=w422, y=w425) -> (0:w430:bool)
          n172 = local write "Refresh Time (ms)"(w418) -> ()
          n173 = call-poly <userlib>:"MGI Wait.vi"("ms"=u32 100, "Error In"=w419) -> ()  [unwired: 5 in, 1 out]
          n174 = local write "Horizontal Progress Bar"(w428) -> ()
          n175 = local write "Delay (ps)"(w428) -> ()
        }
        n176 = call <vilib>:"Add State(s) to Queue__jki_lib_state_machine.vi"("State(s) in (\"\")"=w417) -> ("States Out"=w416:string)  [unwired: 14 in]
      }
      frame "---------- Action ----------" {
        # "Do not put any code in this frame.\n(It is a separator no-op. You can make a copy of this frame to create a new Macro frame)"
        n177 = call <vilib>:"Add State(s) to Queue__jki_lib_state_machine.vi"("State(s) in (\"\")"=w436) -> ("States Out"=w435:string)  [unwired: 14 in]
      }
      frame "Action: Lockin" {
        # "Do not put any code in this frame.\n(It is a separator no-op. You can make a copy of this frame to create a new Macro frame)"
        n178 = Unbundle By Name(w439) -> ("Instruments.DAQ"=w442:refnum<class "Instrument.LockinAPI.lvclass">)
        n179 = case shown="\"Start\", Default" w443 {
          tunnel: w442 -> [w447 w452]
          tunnel: w441 -> [w449 w453]
          tunnel: [w448 w451] -> w440
          tunnel: [w446 w450] -> w438
          frame "Stop" {
            n180 = call-dynamic "waitStatusIdle.vi"("error in (no error)"=w449, "Instrument.LockinAPI in"=w447) -> ("error out"=w448:errorcluster, "Instrument.LockinAPI out"=w446:refnum<class "Instrument.LockinAPI.lvclass">)  [unwired: 8 in]
          }
          frame "Start", Default {
            n181 = call-dynamic "waitStatusSweepingStarted.vi"("error in (no error)"=w453, "Instrument.LockinAPI in"=w452) -> ("error out"=w451:errorcluster, "Instrument.LockinAPI out"=w450:refnum<class "Instrument.LockinAPI.lvclass">)  [unwired: 8 in]
          }
        }
        n182 = Bundle By Name(cluster=w439, "Instruments.DAQ"=w438) -> (w437:T5)
        n183 = call <vilib>:"Add State(s) to Queue__jki_lib_state_machine.vi"("State(s) in (\"\")"=w445) -> ("States Out"=w444:string)  [unwired: 14 in]
      }
      frame "Action: Lockin Sampling" {
        # "#todo: make sure Fs and N are in appropriate range"
        # "Do not put any code in this frame.\n(It is a separator no-op. You can make a copy of this frame to create a new Macro frame)"
        n184 = Unbundle By Name(w456) -> ("Instruments.DAQ"=w463:refnum<class "Instrument.LockinAPI.lvclass">)
        n185 = Multiply(x="Fs (S/s)", y="Lockin Refresh (s)") -> (x*y=w466:dbl)
        n186 = To Long Integer(number=w466) -> (32bit integer=w464:i32)
        n187 = call-dynamic "getSampling.vi"("error in (no error)"=w460, "Instrument.LockinAPI in"=w463) -> ("error out"=w459:errorcluster, "sampling"=w457:T8, "Instrument.LockinAPI out"=w462:refnum<class "Instrument.LockinAPI.lvclass">)  [unwired: 7 in]
        n188 = Bundle By Name(cluster=w457, "Fs"="Fs (S/s)", "#s"=w464) -> (w458:T8)
        n189 = Not Equal?(x=w457, y=w458) -> (x != y?=w461:bool)
        n190 = case shown="True" w461 {
          tunnel: w459 -> [w472 w477]
          tunnel: [w472 w476] -> w468
          tunnel: w462 -> [w471 w475]
          tunnel: w458 -> [_ w474]
          tunnel: [w471 w473] -> w454
          frame False {
          }
          frame True {
            n191 = call-dynamic "setSampling.vi"("error in (no error)"=w477, "sampling"=w474, "Instrument.LockinAPI in"=w475) -> ("error out"=w476:errorcluster, "Instrument.LockinAPI out"=w473:refnum<class "Instrument.LockinAPI.lvclass">)  [unwired: 7 in]
          }
        }
        n192 = Bundle By Name(cluster=w456, "Instruments.DAQ"=w454) -> (w455:T5)
        n193 = call <vilib>:"Add State(s) to Queue__jki_lib_state_machine.vi"("State(s) in (\"\")"=w470) -> ("States Out"=w469:string)  [unwired: 14 in]
      }
      frame "Action: Move Delay Line" {
        # "Do not put any code in this frame.\n(It is a separator no-op. You can make a copy of this frame to create a new Macro frame)"
        n194 = Unbundle By Name(w478) -> ("Instruments.Delay Line"=w487:refnum<class "Instrument.DelayLine.lvclass">, "Delay Speed (ps/s)"=w485:dbl)
        n195 = case shown="\"Start\", Default" w486 {
          tunnel: [w490 w493] -> w483
          tunnel: [1.0 ("Rate (ps/s)") w492] -> w484
          tunnel: w485 -> [_ w492]
          frame "Start", Default {
            n196 = local read "Delay Start (ps)"() -> (w490:dbl)
          }
          frame "End" {
            n197 = local read "Delay End (ps)"() -> (w493:dbl)
          }
        }
        n198 = call-dynamic "setDelay.vi"("error in (no error)"=w482, "Rate (ps/s)"=w484, "Delay (ps)"=w483, "Instrument.Delay in"=w487) -> ("error out"=w481:errorcluster, "Instrument.Delay out"=w480:refnum<class "Instrument.DelayLine.lvclass">)  [unwired: 6 in]
        n199 = Bundle By Name(cluster=w478, "Instruments.Delay Line"=w480) -> (w479:T5)
        n200 = call <vilib>:"Add State(s) to Queue__jki_lib_state_machine.vi"("State(s) in (\"\")"=w489) -> ("States Out"=w488:string)  [unwired: 14 in]
      }
      frame "Action: Close Delay Line" {
        # "Do not put any code in this frame.\n(It is a separator no-op. You can make a copy of this frame to create a new Macro frame)"
        n201 = Unbundle By Name(w496) -> ("Instruments.Delay Line"=w499:refnum<class "Instrument.DelayLine.lvclass">)
        n202 = call-dynamic "Close.vi"("error in (no error)"=w498, "Instrument in"=w499) -> ("error out"=w497:errorcluster, "Instrument out"=w495:refnum<class "Instrument.DelayLine.lvclass">)  [unwired: 8 in]
        n203 = Bundle By Name(cluster=w496, "Instruments.Delay Line"=w495) -> (w494:T5)
        n204 = call <vilib>:"Add State(s) to Queue__jki_lib_state_machine.vi"("State(s) in (\"\")"=w501) -> ("States Out"=w500:string)  [unwired: 14 in]
      }
      frame "---------- Measure ----------" {
        # "Template Separator\n(You can make a copy of, or modify, this frame)"
        n205 = call <vilib>:"Add State(s) to Queue__jki_lib_state_machine.vi"("State(s) in (\"\")"=w505) -> ("States Out"=w504:string)  [unwired: 14 in]
      }
      frame "Measure: Lockin" {
        # "Template Separator\n(You can make a copy of, or modify, this frame)"
        n206 = Unbundle By Name(w516) -> ("t0"=w510:timestamp, "AI Waveform (s)"=w514:waveform(dbl)[], "Instruments.DAQ"=w506:refnum<class "Instrument.LockinAPI.lvclass">)
        n207 = case shown="Default" w508 {
          tunnel: w514 -> [w523 w544]
          tunnel: [w523 w543] -> w513
          tunnel: [w525 w542] -> w512
          tunnel: w509 -> [w526 w541]
          tunnel: [w521 w537] -> w511
          tunnel: w506 -> [w527 w536]
          tunnel: w510 -> [_ w534]
          tunnel: [w519 w533] -> w507
          frame "Start" {
            n208 = for {
              N: 3 -> [_]
              tunnel: [w529] -> w520
              shift-right: [w530] -> w525
              shift-left: w526 -> [w531]
              shift-right: [w528] -> w519
              shift-left: w527 -> [w532]
              n209 = call-dynamic "waitNewWaveforms.vi"("error in (no error)"=w531, "Instrument.LockinAPI in"=w532) -> ("error out"=w530:errorcluster, "Newest AI Waveform"=w529:waveform(dbl)[], "Instrument.LockinAPI out"=w528:refnum<class "Instrument.LockinAPI.lvclass">)  [unwired: 7 in]
            }
            n210 = Index Array(array=w520) -> (element=w524:waveform(dbl))  [unwired: 1 in]
            n211 = Unbundle By Name(w524) -> ("t0"=w521:timestamp)
          }
          frame Default {
            n212 = call-dynamic "getAIwfm.vi"("error in (no error)"=w541, "Instrument.LockinAPI in"=w536) -> ("error out"=w540:errorcluster, "AI Waveform"=w535:waveform(dbl)[], "Instrument.LockinAPI out"=w533:refnum<class "Instrument.LockinAPI.lvclass">)  [unwired: 7 in]
            n213 = Index Array(array=w535) -> (element=w539:waveform(dbl))  [unwired: 1 in]
            n214 = Unbundle By Name(w539) -> ("t0"=w537:timestamp)
            n215 = Equal?(x=w537, y=w534) -> (x = y?=w538:bool)
            n216 = case shown="False" w538 {
              tunnel: w544 -> [w546 w563]
              tunnel: [w549 w563] -> w543
              tunnel: [w548 w564] -> w542
              tunnel: w540 -> [w547 w564]
              tunnel: w535 -> [w550 _]
              frame False {
                n217 = Array Size(array=w546) -> (size(s)=w545:i32)
                n218 = case shown="0" w545 {
                  tunnel: w550 -> [w552 w557]
                  tunnel: [w552 w556] -> w549
                  tunnel: [w551 w555] -> w548
                  tunnel: w547 -> [w551 w554]
                  tunnel: w546 -> [_ w553]
                  frame 0 {
                  }
                  frame Default {
                    n219 = for {
                      tunnel: w553 -> [w558] mode=indexing
                      tunnel: w557 -> [w562] mode=indexing
                      tunnel: [w561] -> w556 mode=indexing
                      tunnel: [w560] -> w555
                      tunnel: w554 -> [w559]
                      n220 = call-poly <vilib>:"Append Waveforms.vi"("error in (no error)"=w559, "waveform B"=w562, "waveform A"=w558) -> ("error out"=w560:errorcluster, "waveform out"=w561:waveform(dbl))  [unwired: 7 in]
                    }
                  }
                }
              }
              frame True {
              }
            }
          }
        }
        n221 = Bundle By Name(cluster=w516, "t0"=w511, "AI Waveform (s)"=w513, "Instruments.DAQ"=w507) -> (w515:T5)
        n222 = call <vilib>:"Add State(s) to Queue__jki_lib_state_machine.vi"("State(s) in (\"\")"=w518) -> ("States Out"=w517:string)  [unwired: 14 in]
      }
      frame "Measure: Temperature" {
        # "Your code here.\n(You can make a copy of, or modify, this frame)"
        n223 = Unbundle By Name(w573) -> ("C.E."=w568:refnum<class "Control Experiment.lvclass">, "Instruments.Temperature"=w575:refnum<class "Instrument.Cryostat.lvclass">)
        n224 = call-dynamic "getTemperature.vi"("error in (no error)"=w574, "Instrument.Cryostat in"=w575) -> ("error out"=w570:errorcluster, "Temperature (K)"=w569:dbl, "Instrument.Cryostat out"=w565:refnum<class "Instrument.Cryostat.lvclass">)  [unwired: 5 in, 2 out]
        "T (mK)" <- w569
        n225 = call "Append Dictionary Element.vi"("error in (no error)"=w570, "value"=w569, "key"="Temperature", "Control Experiment in"=w568) -> ("error out"=w567:errorcluster, "Control Experiment out"=w566:refnum<class "Control Experiment.lvclass">)  [unwired: 6 in]
        n226 = Bundle By Name(cluster=w573, "Instruments.Temperature"=w565, "Temperature"=w569, "C.E."=w566) -> (w572:T5)
        n227 = call <vilib>:"Add State(s) to Queue__jki_lib_state_machine.vi"("State(s) in (\"\")"=w577) -> ("States Out"=w576:string)  [unwired: 14 in]
      }
      frame "Measure: Time" {
        # "Your code here.\n(You can make a copy of, or modify, this frame)"
        n228 = Unbundle By Name(w596) -> ("reset"=w580:bool, "Elapsed Time"=w590:dbl[], "Absolute Time"=w584:dbl[], "C.E."=w594:refnum<class "Control Experiment.lvclass">)
        n229 = Get Date/Time In Seconds() -> (seconds since 1Jan1904=w586:timestamp)
        n230 = Select(t=2, s=w580, f=1) -> (s? t:f=w581:i32)
        n231 = for {
          N: w581 -> [_]
          tunnel: [w601] -> w588
          tunnel: w580 -> [w600]
          n232 = call <userlib>:"MGI Milliseconds Since Last Reset.vi"("Reset (F)"=w600) -> ("ms"=w601:u32)  [unwired: 5 in, 1 out]
        }
        n233 = To Double Precision Float(number=w586) -> (double precision float=w583:dbl)
        n234 = Divide(x=w588, y=u32 1000) -> (x/y=w587:dbl)
        n235 = call "Append Dictionary Element.vi"("error in (no error)"=w592, "value"=w583, "key"="Time", "Control Experiment in"=w594) -> ("error out"=w591:errorcluster, "Control Experiment out"=w595:refnum<class "Control Experiment.lvclass">)  [unwired: 6 in]
        n236 = Build Array (concatenate)(w584, w583) -> (w585:dbl[])
        n237 = Build Array (concatenate)(w590, w587) -> (w589:dbl[])
        n238 = Bundle By Name(cluster=w596, "Elapsed Time"=w589, "Absolute Time"=w585, "C.E."=w595) -> (w597:T5)
        n239 = call <vilib>:"Add State(s) to Queue__jki_lib_state_machine.vi"("State(s) in (\"\")"=w599) -> ("States Out"=w598:string)  [unwired: 14 in]
      }
      frame "Measure: Delay Line" {
        # "Template Separator\n(You can make a copy of, or modify, this frame)"
        n240 = Unbundle By Name(w615) -> ("Delay"=w609:dbl[], "C.E."=w610:refnum<class "Control Experiment.lvclass">, "Instruments.Delay Line"=w613:refnum<class "Instrument.DelayLine.lvclass">)
        n241 = call-dynamic "getDelay.vi"("error in (no error)"=w607, "Instrument.DelayLine in"=w613) -> ("error out"=w611:errorcluster, "delay (ps)"=w602:dbl, "Instrument.DelayLine out"=w603:refnum<class "Instrument.DelayLine.lvclass">, "Finished?"=w604:bool)  [unwired: 6 in]
        "Delay (ps)" <- w602
        "Horizontal Progress Bar" <- w602
        n242 = Build Array (concatenate)(w609, w602) -> (w608:dbl[])
        n243 = call "Append Dictionary Element.vi"("error in (no error)"=w611, "value"=w602, "key"="Delay", "Control Experiment in"=w610) -> ("error out"=w606:errorcluster, "Control Experiment out"=w612:refnum<class "Control Experiment.lvclass">)  [unwired: 6 in]
        n244 = Bundle By Name(cluster=w615, "Delay"=w608, "Instruments.Delay Line"=w603, "C.E."=w612, "delay line finish?"=w604) -> (w614:T5)
        n245 = call <vilib>:"Add State(s) to Queue__jki_lib_state_machine.vi"("State(s) in (\"\")"=w617) -> ("States Out"=w616:string)  [unwired: 14 in]
      }
      frame "---------- File ----------" {
        # "Template Separator\n(You can make a copy of, or modify, this frame)"
        n246 = call <vilib>:"Add State(s) to Queue__jki_lib_state_machine.vi"("State(s) in (\"\")"=w621) -> ("States Out"=w620:string)  [unwired: 14 in]
      }
      frame "File: Configure" {
        # "Template Separator\n(You can make a copy of, or modify, this frame)"
        n247 = call <vilib>:"Add State(s) to Queue__jki_lib_state_machine.vi"("State(s) in (\"\")"=w625) -> ("States Out"=w624:string)  [unwired: 14 in]
      }
      frame "File: Save" {
        # "Template Separator\n(You can make a copy of, or modify, this frame)"
        n248 = Unbundle By Name(w629) -> ("Execution:State"=w630:T6, "C.E."=w631:refnum<class "Control Experiment.lvclass">, "AI Waveform (ps)"=w632:waveform(dbl)[])
        n249 = for {
          tunnel: w631 -> [w675]
          tunnel: [w674] -> w637
          tunnel: [w673] -> w636
          tunnel: w634 -> [w658]
          tunnel: w632 -> [w653] mode=indexing
          tunnel: w634 -> [w647]
          tunnel: [w640] -> w633 mode=indexing
          i -> [w680]
          n250 = call-poly <vilib>:"Waveform to XY.vi"("error in (no error)"=w647, "Waveform in"=w653) -> ("error out"=w648:errorcluster, "XY-data out"=w651:cluster{"X-array":dbl[], "Y-array":dbl[]})  [unwired: 8 in]
          n251 = call-poly <vilib>:"FFT Power Spectrum and PSD.vi"("error in (no error)"=w647, "time signal"=w653) -> ("error out"=w642:errorcluster, "Power Spectrum / PSD"=w640:cluster{"f0":dbl, "df":dbl, "magnitude":dbl[]})  [unwired: 6 in, 2 out]
          n252 = Increment(x=w680) -> (x+1=w678:i32)
          n253 = call-poly <vilib>:"Get X and Y.vi"("error in (no error)"=w648, "XY-data"=w651) -> ("Y-array"=w649:dbl[], "X-array"=w650:dbl[])  [unwired: 6 in, 2 out]
          n254 = Format Into String(format string="Ch%d" ("wavenames"), w678) -> (resulting string=w659:string)  [unwired: 2 in, 1 out]
          n255 = Unbundle By Name(w640) -> ("f0"=w657:dbl, "df"=w656:dbl, "magnitude"=w655:dbl[])
          n256 = Concatenate Strings(w659, "_x" ("string")) -> (w667:string)
          n257 = call "Write Dictionary Element.vi"("error in (no error)"=w658, "value"=w650, "key"=w667, "Control Experiment in"=w675) -> ("error out"=w671:errorcluster, "Control Experiment out"=w672:refnum<class "Control Experiment.lvclass">)  [unwired: 6 in]
          n258 = To Time Stamp(1:w657) -> (0:w654:timestamp)
          n259 = Concatenate Strings(w659, "_y" ("string")) -> (w665:string)
          n260 = Bundle By Name("t0"=w654, "dt"=w656, "Y"=w655) -> (w641:waveform(dbl))  [unwired: 1 in]
          n261 = call "Write Dictionary Element.vi"("error in (no error)"=w671, "value"=w649, "key"=w665, "Control Experiment in"=w672) -> ("error out"=w652:errorcluster, "Control Experiment out"=w677:refnum<class "Control Experiment.lvclass">)  [unwired: 6 in]
          n262 = Concatenate Strings(w659, "_PS" ("string")) -> (w662:string)
          n263 = call-poly <vilib>:"Waveform to XY.vi"("error in (no error)"=w642, "Waveform in"=w641) -> ("error out"=w646:errorcluster, "XY-data out"=w645:cluster{"X-array":dbl[], "Y-array":dbl[]})  [unwired: 8 in]
          n264 = call-poly <vilib>:"Get X and Y.vi"("error in (no error)"=w646, "XY-data"=w645) -> ("Y-array"=w643:dbl[], "X-array"=w644:dbl[])  [unwired: 6 in, 2 out]
          n265 = Concatenate Strings(w662, "_x" ("string")) -> (w661:string)
          n266 = call "Write Dictionary Element.vi"("error in (no error)"=w652, "value"=w644, "key"=w661, "Control Experiment in"=w677) -> ("error out"=w669:errorcluster, "Control Experiment out"=w670:refnum<class "Control Experiment.lvclass">)  [unwired: 6 in]
          n267 = Concatenate Strings(w662, "_y" ("string")) -> (w660:string)
          n268 = call "Write Dictionary Element.vi"("error in (no error)"=w669, "value"=w643, "key"=w660, "Control Experiment in"=w670) -> ("error out"=w673:errorcluster, "Control Experiment out"=w674:refnum<class "Control Experiment.lvclass">)  [unwired: 6 in]
        }
        "Power Spectrum" <- w633
        n269 = call "Exec State to Append.vi"("Execution:State"=w630) -> ()  [unwired: 2 in, 1 out]
        n270 = call "Save Transport TDMS File.vi"("append?"=FALSE, "error in (no error)"=w636, "Control Experiment in"=w637) -> ("error out"=w635:errorcluster, "Control Experiment out"=w627:refnum<class "Control Experiment.lvclass">)  [unwired: 7 in]
        n271 = Bundle By Name(cluster=w629, "C.E."=w627) -> (w628:T5)
        n272 = call <vilib>:"Add State(s) to Queue__jki_lib_state_machine.vi"("State(s) in (\"\")"=w639) -> ("States Out"=w638:string)  [unwired: 14 in]
      }
      frame "File: JSON" {
        # "#todo: add save JSON stuff"
        # "Template Separator\n(You can make a copy of, or modify, this frame)"
        n273 = Unbundle By Name(w682) -> ()  [unwired: 1 out]
        n274 = call <vilib>:"Add State(s) to Queue__jki_lib_state_machine.vi"("State(s) in (\"\")"=w684) -> ("States Out"=w683:string)  [unwired: 14 in]
      }
    }
  }
  "error out" <- w3
  n275 = Unbundle By Name(w4) -> ("Transport"=→"Transport out":refnum<class "Transport.lvclass">)
